vi "Configure Linear Calculation.vi"(7 "mX+b Units (MXB)":string="MXB", 8 "error in (no error)":errorcluster, 9 "Offset (b) Value (0.000000)":dbl, 10 "Scale Factor (m) Value (1.000000)":dbl=1.0, 11 "VISA resource name":refnum<visa-resource-name>) -> (0 "error out":errorcluster, 3 "VISA resource name out":refnum<visa-resource-name>)   [LabVIEW 2019, in "Keithley 6517.lvlib"]
doc: "Configures the mX+b calculation for model 6514.\n\n<B>Note:</B>\nThis VI is ONLY comparible with <B>model 6514</B>. Running this VI with any other model will result in an error."
uses:
  Keithley 6517.lvlib
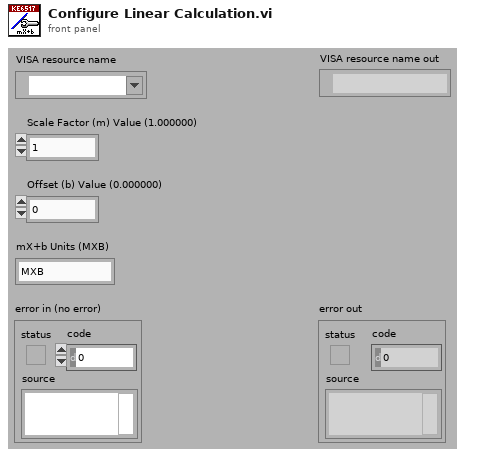
[diagram p1: front panel]
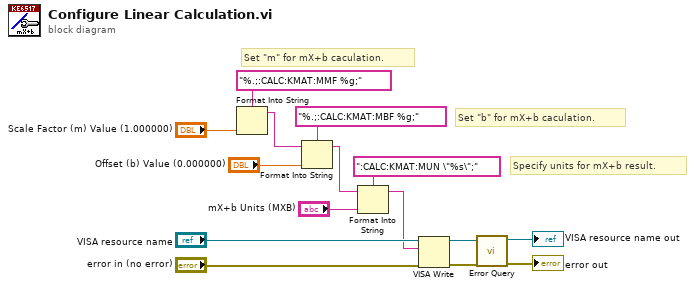
[diagram p0: block diagram]
diagram:
  # "Set \"m\" for mX+b caculation."
  # "Specify units for mX+b result."
  # "Set \"b\" for mX+b caculation."
  n1 = Format Into String(format string="%.;:CALC:KMAT:MMF %g;", "Scale Factor (m) Value (1.000000)") -> (resulting string=w4:string)  [unwired: 2 in, 1 out]
  n2 = Format Into String(format string="%.;:CALC:KMAT:MBF %g;", initial string=w4, "Offset (b) Value (0.000000)") -> (resulting string=w5:string)  [unwired: 1 in, 1 out]
  n3 = Format Into String(format string=":CALC:KMAT:MUN \"%s\";" ("command"), initial string=w5, "mX+b Units (MXB)") -> (resulting string=w1:string)  [unwired: 1 in, 1 out]
  n4 = VISA Write(VISA resource name="VISA resource name", write buffer=w1, error in (no error)="error in (no error)") -> (VISA resource name out=w11:refnum<visa-resource-name>, error out=w12:errorcluster)  [unwired: 1 out]
  n5 = call "Error Query.vi"("error in (no error)"=w12, "VISA resource name"=w11) -> ("error out"=→"error out":errorcluster, "VISA resource name out"=→"VISA resource name out":refnum<visa-resource-name>)  [unwired: 6 in, 2 out]
